vi "ConfigureChannelsForMCSA(60s).vi"(6 "supported metrics":string[](array[string]), 8 "error in (no error)":errorcluster, 9 "metric cache":variant, 11 "device":T5) -> (0 "error out":errorcluster, 2 "Motor":T1, 3 "channels":T2[](array[typedef]))   [LabVIEW 2017, in "McsaAnalysisFunctions.lvlib"]
uses:
  <vilib>/addons/InsightCM/Utilities/Analysis/MCSA/McsaAnalysisFunctions.lvlib
  <vilib>/addons/InsightCM/MessageBus/Base/controls/R2_DeviceModel.ctl
  <vilib>/addons/InsightCM/MessageBus/Base/controls/R2_Device.ctl
  <vilib>/addons/InsightCM/MessageBus/Base/controls/KeyValuePair.ctl
  <vilib>/addons/InsightCM/MessageBus/Base/controls/DeviceState.ctl
  <vilib>/addons/InsightCM/MessageBus/Base/controls/R2_DataGroup.ctl
  <vilib>/addons/InsightCM/MessageBus/Base/controls/OperatingState.ctl
  <vilib>/addons/InsightCM/MessageBus/Base/controls/Trigger.ctl
  <vilib>/addons/InsightCM/MessageBus/Base/controls/Condition.ctl
  <vilib>/addons/InsightCM/MessageBus/Base/controls/BurstModeTrigger.ctl
  <vilib>/addons/InsightCM/MessageBus/Base/controls/R2_Channel.ctl
  <vilib>/addons/InsightCM/MessageBus/Base/controls/Metric.ctl
  <vilib>/addons/InsightCM/MessageBus/Base/controls/Tag.ctl
  <vilib>/addons/InsightCM/Utilities/Analysis/MCSA/controls/McsaLowUpdateChannel.ctl
  <vilib>/addons/InsightCM/Utilities/Analysis/Shared/controls/Feature.ctl
  <vilib>/addons/InsightCM/Utilities/Analysis/Shared/controls/AmplitudeScale.ctl
  <vilib>/addons/InsightCM/Utilities/Analysis/MCSA/controls/McsaMotor.ctl
  <vilib>/addons/InsightCM/Utilities/PropertyHelpers/PropertyHelpers.lvlib
  <vilib>/addons/InsightCM/Utilities/Analysis/Shared/AnalysisHelper.lvlib
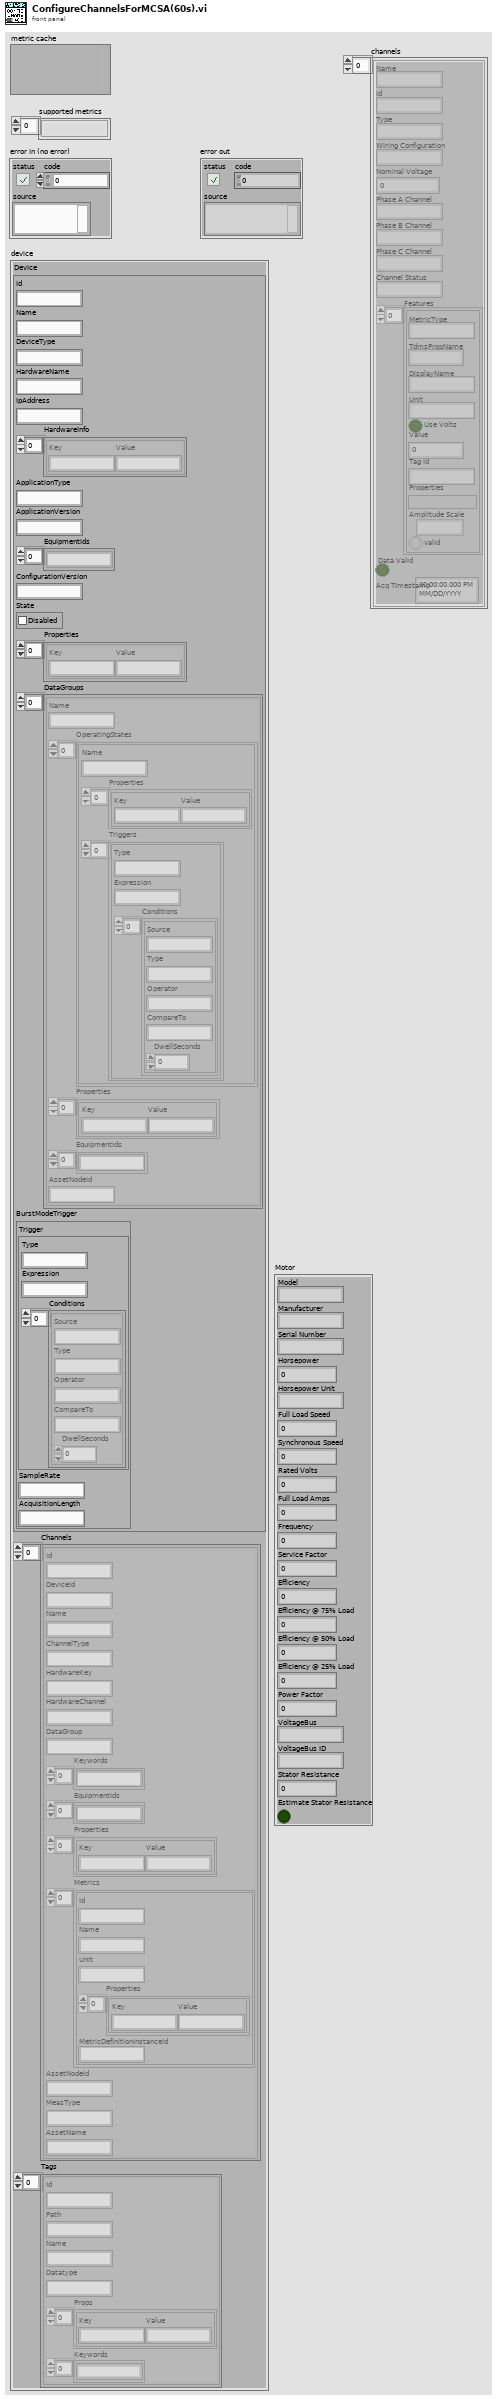
[diagram p1: front panel]
types:
  T1 = typedef "McsaAnalysisFunctions.lvlib/McsaMotor.ctl" = cluster{"Model":string, "Manufacturer":string, "Serial Number":string, "Horsepower":dbl, "Horsepower Unit":string, "Full Load Speed":dbl, "Synchronous Speed":dbl, "Rated Volts":dbl, "Full Load Amps":dbl, "Frequency":dbl, "Service Factor":dbl, "Efficiency":dbl, "Efficiency @ 75% Load":dbl, "Efficiency @ 50% Load":dbl, "Efficiency @ 25% Load":dbl, "Power Factor":dbl, "VoltageBus":string, "VoltageBus ID":string, "Stator Resistance":dbl, "Estimate Stator Resistance":bool}
  T2 = typedef "McsaAnalysisFunctions.lvlib/McsaLowUpdateChannel.ctl" = cluster{"Name":string, "Id":string, "Type":string, "Wiring Configuration":string, "Nominal Voltage":dbl, "Phase A Channel":string, "Phase B Channel":string, "Phase C Channel":string, "Channel Status":string, "Features":T3[], "Data Valid":bool, "Acq Timestamp":timestamp}
  T3 = typedef "AnalysisHelper.lvlib/Feature.ctl" = cluster{"MetricType":string, "TdmsPropName":string, "DisplayName":string, "Unit":string, "Use Volts":bool, "Value":dbl, "Tag Id":string, "Properties":variant, "Amplitude Scale":T4, "valid":bool}
  T4 = typedef "AnalysisHelper.lvlib/AmplitudeScale.ctl" = enum16{"rms", "peak", "pk-pk"}
  T5 = typedef "R2_DeviceModel.ctl" = cluster{"Device":T6, "Channels":T14[], "Tags":T16[]}
  T6 = typedef "R2_Device.ctl" = cluster{"Id":string, "Name":string, "DeviceType":string, "HardwareName":string, "IpAddress":string, "HardwareInfo":T7[], "ApplicationType":string, "ApplicationVersion":string, "EquipmentIds":string[], "ConfigurationVersion":string, "State":T8, "Properties":T7[], "DataGroups":T9[], "BurstModeTrigger":T13}
  T7 = typedef "KeyValuePair.ctl" = cluster{"Key":string, "Value":string}
  T8 = typedef "DeviceState.ctl" = cluster{"Disabled":bool}
  T9 = typedef "R2_DataGroup.ctl" = cluster{"Name":string, "OperatingStates":T10[], "Properties":T7[], "EquipmentIds":string[], "AssetNodeId":string}
  T10 = typedef "OperatingState.ctl" = cluster{"Name":string, "Properties":T7[], "Triggers":T11[]}
  T11 = typedef "Trigger.ctl" = cluster{"Type":string, "Expression":string, "Conditions":T12[]}
  T12 = typedef "Condition.ctl" = cluster{"Source":string, "Type":string, "Operator":string, "CompareTo":string, "DwellSeconds":dbl}
  T13 = typedef "BurstModeTrigger.ctl" = cluster{"Trigger":T11, "SampleRate":string, "AcquisitionLength":string}
  T14 = typedef "R2_Channel.ctl" = cluster{"Id":string, "DeviceId":string, "Name":string, "ChannelType":string, "HardwareKey":string, "HardwareChannel":string, "DataGroup":string, "Keywords":string[], "EquipmentIds":string[], "Properties":T7[], "Metrics":T15[], "AssetNodeId":string, "MeasType":string, "AssetName":string}
  T15 = typedef "Metric.ctl" = cluster{"Id":string, "Name":string, "Unit":string, "Properties":T7[], "MetricDefinitionInstanceId":string}
  T16 = typedef "Tag.ctl" = cluster{"Id":string, "Path":string, "Name":string, "Datatype":string, "Props":T7[], "Keywords":string[]}
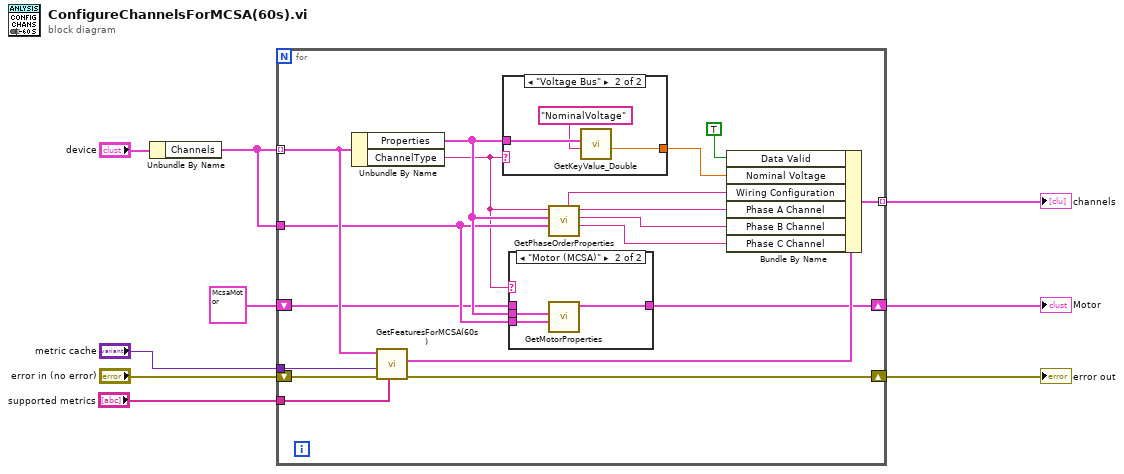
[diagram p0: block diagram]
diagram:
  n1 = Unbundle By Name("device") -> ("Channels"=w4:T14[])
  n2 = for {
    tunnel: [w24] -> w3 mode=indexing
    tunnel: "metric cache" -> [w26]
    tunnel: w4 -> [w25] mode=indexing
    shift-right: [w21] -> w6
    shift-left: "error in (no error)" -> [w27]
    tunnel: w4 -> [w17]
    tunnel: "supported metrics" -> [w23]
    shift-right: [w12] -> w2
    shift-left: T1 {"Model"="", "Manufacturer"="", "Serial Number"="", "Horsepower"=0.0, "Horsepower Unit"="", "Full Load Speed"=0.0, "Synchronous Speed"=0.0, "Rated Volts"=0.0, "Full Load Amps"=0.0, "Frequency"=0.0, "Service Factor"=0.0, "Efficiency"=0.0, "Efficiency @ 75% Load"=0.0, "Efficiency @ 50% Load"=0.0, "Efficiency @ 25% Load"=0.0, "Power Factor"=0.0, "VoltageBus"="", "VoltageBus ID"="", "Stator Resistance"=0.0, "Estimate Stator Resistance"=FALSE} ("Motor") -> [w10]
    n3 = Unbundle By Name(w25) -> ("Properties"=w18:T7[], "ChannelType"=w11:string)
    n4 = call <vilib>:"GetFeaturesForMCSA(60s).vi"("supported features"=w23, "error in (no error)"=w27, "Metric Cache"=w26, "ChannelModel"=w25) -> ("error out"=w21:errorcluster, "channels"=w22:T2)  [unwired: 6 in]
    n5 = case shown="\"Voltage Bus\"" w11 {
      tunnel: w18 -> [_ w34]
      tunnel: [_ w32] -> w20
      frame Default {
      }
      frame "Voltage Bus" {
        n6 = call <vilib>:"GetKeyValue_Double.vi"("key"="NominalVoltage", "key value pairs"=w34) -> ("value"=w32:dbl)  [unwired: 7 in, 2 out]
      }
    }
    n7 = case shown="\"Motor (MCSA)\"" w11 {
      tunnel: w18 -> [_ w31]
      tunnel: w17 -> [_ w30]
      tunnel: [w28 w29] -> w12
      tunnel: w10 -> [w28 _]
      frame Default {
      }
      frame "Motor (MCSA)" {
        n8 = call <vilib>:"GetMotorProperties.vi"("Channels"=w30, "Channel Properties"=w31) -> ("Motor"=w29:T1)  [unwired: 7 in, 2 out]
      }
    }
    n9 = call <vilib>:"GetPhaseOrderProperties.vi"("Channels"=w17, "Channel Properties"=w18, "ChannelType"=w11) -> ("Phase C ChannelName"=w14:string, "Phase B ChannelName"=w15:string, "Phase A ChannelName"=w16:string, "wiring configuraiton"=w19:string)  [unwired: 4 in, 1 out]
    n10 = Bundle By Name(cluster=w22, "Data Valid"=TRUE, "Nominal Voltage"=w20, "Wiring Configuration"=w19, "Phase A Channel"=w16, "Phase B Channel"=w15, "Phase C Channel"=w14) -> (w24:T2)
  }
  "channels" <- w3
  "error out" <- w6
  "Motor" <- w2
